vi "Simple DataSocket - Writer.vi"() -> ()   [LabVIEW 2019]
doc: "Uses DataSocket to write array data. This example works for writing the data to the DataSocket Server (for live data). \n \nThe Writer, Server, and Reader can all be on the same computer or different computers. The Writer and Reader URLs should point to the computer where the DataSocket Server is."
panel:
  in  "Stop":bool
  out "Data Written":dbl[](graph)
  # "Overview: Demonstrates the use of the DataSocket functions to write data to the DataSocket server.\nRequirements: Windows\nInstructions:\n1. Run the DataSocket server by navigating the Windows start menu to National Instruments > DataSocket > DataSocket Server.\n2. Run the VI.\n3. Open Simple DataSocket - Reader.vi and follow the instructions on its front panel.\n4. Click Stop to stop the VI."
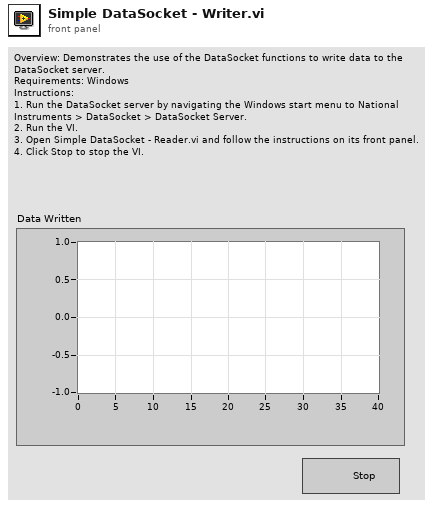
[diagram p1: front panel]
types:
  T1 = enum16{"Read", "Write", "ReadWrite", "BufferedRead", "BufferedReadWrite"}
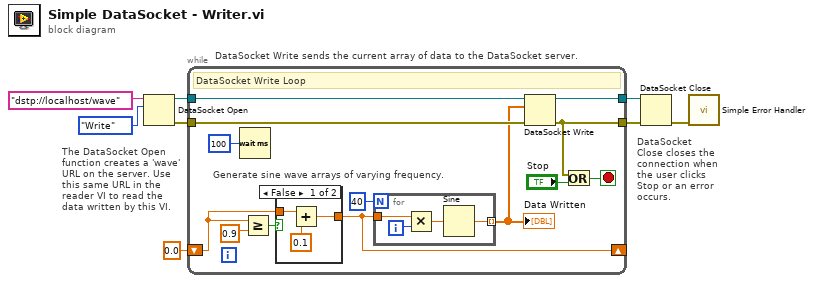
[diagram p0: block diagram]
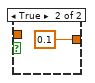
[diagram p2: hidden frame]
diagram:
  # "The DataSocket Open function creates a 'wave' URL on the server. Use this same URL in the reader VI to read the data written by this VI."
  # "DataSocket Write sends the current array of data to the DataSocket server."
  # "DataSocket Close closes the connection when the user clicks Stop or an error occurs."
  n1 = DataSocket Open(10:T1."Write" ("mode"), 11:"dstp://localhost/wave" ("Write Location")) -> (0:w5:errorcluster, 3:w6:refnum<k13>)  [unwired: 2 in]
  n2 = while {
    shift-left: 0.0 -> [w17]
    shift-right: [w16] -> _
    tunnel: [w12] -> w8
    tunnel: w6 -> [w20]
    tunnel: w5 -> [w21]
    tunnel: [w9] -> w3
    stop <- w18 stop-if-true
    # "Generate sine wave arrays of varying frequency."
    # "DataSocket Write Loop"
    n3 = Wait (ms)(milliseconds to wait=u32 100) -> ()  [unwired: 1 out]
    n4 = Greater Or Equal?(x=w17, y=0.9) -> (x >= y?=w13:bool)
    n5 = case shown="False" w13 {
      tunnel: [w27 0.1] -> w16
      tunnel: w17 -> [w28 _]
      frame False {
        n6 = Add(x=w28, y=0.1) -> (x+y=w27:dbl)
      }
      frame True {
      }
    }
    n7 = for {
      N: 40 -> [_]
      tunnel: w16 -> [w25]
      tunnel: [w22] -> w10 mode=indexing
      i -> [w24]
      n8 = Multiply(x=w25, y=w24) -> (x*y=w23:dbl)
      n9 = Sine(x=w23) -> (sin(x)=w22:dbl)
    }
    "Data Written" <- w10
    n10 = DataSocket Write(8:w21, 10:w10, 11:w20) -> (0:w12:errorcluster, 3:w9:refnum<k13>)  [unwired: 2 out]
    n11 = Or(x=w12, y="Stop") -> (x .or. y?=w18:bool)
  }
  n12 = DataSocket Close(8:w8, 11:w3) -> (0:w4:errorcluster)  [unwired: 1 in, 1 out]
  n13 = call <vilib>:"Simple Error Handler.vi"("error in (no error)"=w4) -> ()  [unwired: 4 in, 5 out]
